vi "Init - Add Events.vi"(8 "error in (no error)":errorcluster, 10 "ECUEvent Components":T2[](array[typedef]), 11 "Device ref in":T1 format="%.0x") -> (0 "error out":errorcluster, 3 "Device ref out":T1 format="%.0x")   [LabVIEW 2011, in "Engine Sim System Explorer.lvlib"]
uses:
  Engine Sim System Explorer.lvlib
  TypeDefs/ECUEventComp.ctl
  <vilib>/NI Veristand/Custom Device API/Custom Device Item Ref.ctl
  <vilib>/NI Veristand/Custom Device API/Custom Device Channel.ctl
  <vilib>/NI Veristand/Custom Device API/Custom Device Channel Type.ctl
  Shared/Engine Simulation Global.vi
  <vilib>/NI Veristand/Custom Device API/Custom Device API.lvlib
  Engine Simulation Shared.lvlib
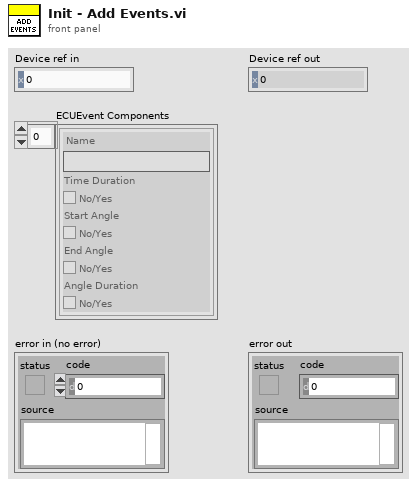
[diagram p1: front panel]
types:
  T1 = typedef "Custom Device API.lvlib/Custom Device Item Ref.ctl" = u64
  T2 = typedef "Engine Sim System Explorer.lvlib/ECUEventComp.ctl" = cluster{"Name":string, "Time Duration":bool, "Start Angle":bool, "End Angle":bool, "Angle Duration":bool}
  T3 = typedef "Custom Device API.lvlib/Custom Device Channel.ctl" = cluster{"Type":T4, "Units":string, "Default Value":dbl, "Faultable":bool, "Scalable":bool}
  T4 = typedef "Custom Device API.lvlib/Custom Device Channel Type.ctl" = enum16{"Input", "Output"}
  T5 = cluster{"Time Duration":bool, "Start Angle":bool, "End Angle":bool, "Angle Duration":bool}
  T6 = cluster{"Time Duration":bool, "Start Angle":bool, "End Angle":bool, "Angle Duration":bool}[]
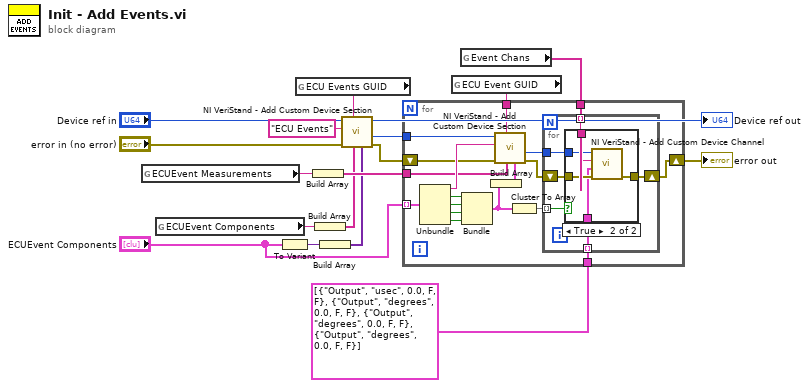
[diagram p0: block diagram]
diagram:
  n1 = global read "Engine Simulation Global.vi" "ECUEvent Measurements"() -> (w17:string)
  n2 = global read "Engine Simulation Global.vi" "ECUEvent Components"() -> (w9:string)
  n3 = To Variant(anything="ECUEvent Components") -> (Variant=w6:variant)
  n4 = global read "Engine Simulation Global.vi" "ECU Events GUID"() -> (w3:string)
  n5 = Build Array(w17) -> (w18:string[])
  n6 = Build Array(w9) -> (w8:string[])
  n7 = Build Array(w6) -> (w7:variant[])
  n8 = call <vilib>:"NI VeriStand - Add Custom Device Section.vi"("Property Values"=w7, "Property names"=w8, "GUID (Default Section)"=w3, "error in (no error)"="error in (no error)", "Section Name"="ECU Events", "Parent Ref in"="Device ref in") -> ("error out"=w13:errorcluster, "Section Ptr"=w11:T1, "Parent Ref out"=→"Device ref out":T1)  [unwired: 2 in, 1 out]
  n9 = global read "Engine Simulation Global.vi" "ECU Event GUID"() -> (w16:string)
  n10 = global read "Engine Simulation Global.vi" "Event Chans"() -> (w1:string[])
  n11 = for {
    tunnel: w11 -> [w35]
    tunnel: "ECUEvent Components" -> [w36] mode=indexing
    shift-right: [w24] -> w15
    shift-left: w13 -> [w33]
    tunnel: w1 -> [w26]
    tunnel: T3[] [{"Type"=enum."Output", "Units"="usec", "Default Value"=0.0, "Faultable"=FALSE, "Scalable"=FALSE}, {"Type"=enum."Output", "Units"="degrees", "Default Value"=0.0, "Faultable"=FALSE, "Scalable"=FALSE}, {"Type"=enum."Output", "Units"="degrees", "Default Value"=0.0, "Faultable"=FALSE, "Scalable"=FALSE}, {"Type"=enum."Output", "Units"="degrees", "Default Value"=0.0, "Faultable"=FALSE, "Scalable"=FALSE}] -> [w25]
    tunnel: w16 -> [w23]
    tunnel: w18 -> [w19]
    n12 = Unbundle(w36) -> ("Name"=w34:string, "Time Duration"=w27:bool, "Start Angle"=w28:bool, "End Angle"=w29:bool, "Angle Duration"=w30:bool)
    n13 = Bundle("Time Duration"=w27, "Start Angle"=w28, "End Angle"=w29, "Angle Duration"=w30) -> (w21:T5)  [unwired: 1 in]
    n14 = Build Array(w21) -> (w20:T6)
    n15 = call <vilib>:"NI VeriStand - Add Custom Device Section.vi"("Property Values"=w20, "Property names"=w19, "GUID (Default Section)"=w23, "error in (no error)"=w33, "Section Name"=w34, "Parent Ref in"=w35) -> ("error out"=w32:errorcluster, "Section Ptr"=w31:T1)  [unwired: 2 in, 2 out]
    n16 = Cluster To Array(cluster=w21) -> (array=w22:bool[])
    n17 = for {
      tunnel: w31 -> [w41]
      shift-right: [w37] -> w24
      shift-left: w32 -> [w42]
      tunnel: w22 -> [w40] mode=indexing
      tunnel: w26 -> [w39] mode=indexing
      tunnel: w25 -> [w38] mode=indexing
      n18 = case shown="True" w40 {
        tunnel: w42 -> [w43 w48]
        tunnel: w41 -> [_ w47]
        tunnel: w39 -> [_ w46]
        tunnel: w38 -> [_ w45]
        tunnel: [w43 w44] -> w37
        frame False {
        }
        frame True {
          n19 = call <vilib>:"NI VeriStand - Add Custom Device Channel.vi"("error in (no error)"=w48, "Channel"=w45, "Channel Name"=w46, "Parent Ref in"=w47) -> ("error out"=w44:errorcluster)  [unwired: 4 in, 3 out]
        }
      }
    }
  }
  "error out" <- w15
